vi "checkFinishDeadBallPlayVSS.vi"(8 "error in (no error)":errorcluster, 9 "last command_interpreted":T1, 10 "Game":refnum<class "Game.lvclass">, 11 "DeadBallPlayVSS in":refnum<class "DeadBallPlayVSS.lvclass">) -> (0 "error out":errorcluster, 2 "Boolean":bool, 3 "DeadBallPlayVSS out":refnum<class "DeadBallPlayVSS.lvclass">)   [LabVIEW 2023, in "DeadBallPlayVSS.lvclass"]
uses:
  DeadBallPlayVSS.lvclass
  Game_class/Game.lvclass
  Referee_class/command_interpreted.ctl
  Utilities_class/Utilities.lvclass
  Game_class/Game.lvclass/Game.ctl
  Ball_class/Ball.lvclass/Ball.ctl
  Events_class/Events.lvclass/Events.ctl
  Game_class/Read BallRef.vi
  Game_class/Read EventsRef.vi
  Events_class/Read ball_out.vi
  Events_class/Read ball_out_of_vision.vi
  Ball_class/Read v_x.vi
  Ball_class/Read v_y.vi
  Ball_class/Ball.lvclass
  Events_class/Events.lvclass
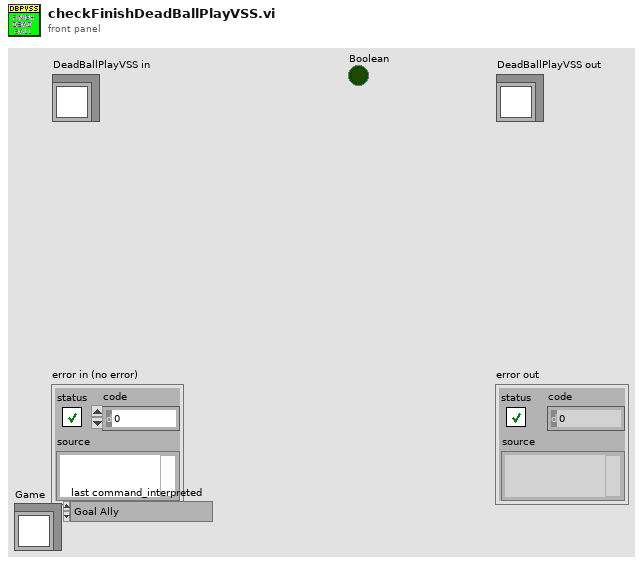
[diagram p1: front panel]
types:
  T1 = typedef "command_interpreted.ctl" = enum16{"Goal Ally", "Goal Enemy", "Ball Placement Enemy", "Ball Placement Ally", "Normal Half Time", "Extra Time  Break", "Extra Half Time", "None", "Post Game", "PKA Normal Start", "Prepare Kickoff Ally", "PKE Normal Start", "Prepare Kickoff Enemy", "Force Start", "Halt", "Timeout", "Prepare Penalty Ally", "Prepare Penalty Enemy", "PPA NormalStart", "PPE Normal Start", "Indirect Free Ally", "Direct Free Enemy", "Direct Free Ally", "Indirect Free Enemy", "Stop"}
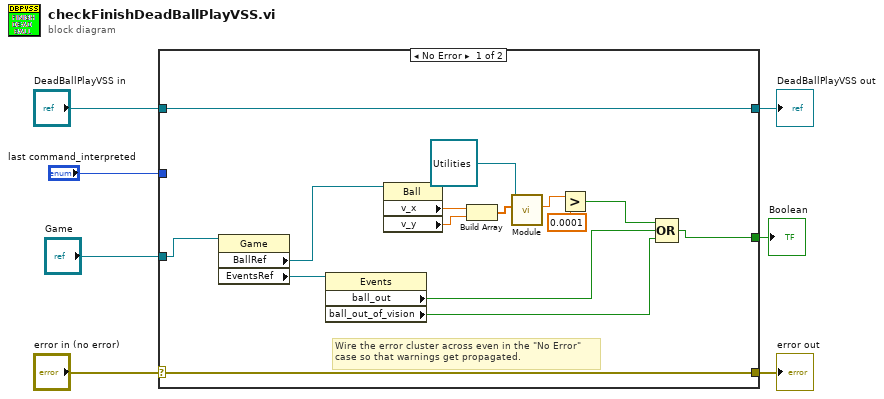
[diagram p0: block diagram]
diagram:
  n1 = case shown="No Error" "error in (no error)" {
    selector: "error in (no error)" -> [w21 w24]
    tunnel: [w21 w24] -> w6
    tunnel: [w22 w23] -> w4
    tunnel: "DeadBallPlayVSS in" -> [w22 w23]
    tunnel: "last command_interpreted" -> [_ _]
    tunnel: "Game" -> [w20 _]
    tunnel: [w8 _] -> w1
    frame No Error {
      # "Wire the error cluster across even in the \"No Error\"\ncase so that warnings get propagated."
      n2 = property class="Game"(reference=w20) -> ("BallRef"=w19:refnum<class "Ball.lvclass">, "EventsRef"=w12:refnum<class "Events.lvclass">)  [unwired: 1 in, 2 out]
      n3 = property class="Events"(reference=w12) -> ("ball_out"=w10:bool, "ball_out_of_vision"=w9:bool)  [unwired: 1 in, 2 out]
      n4 = property class="Ball"(reference=w19) -> ("v_x"=w18:dbl, "v_y"=w17:dbl)  [unwired: 1 in, 2 out]
      n5 = Build Array(w18, w17) -> (w16:dbl[])
      n6 = call-dynamic "Module.vi"("2D vector"=w16, "Utilities in"=refnum<class "Utilities.lvclass"> refnum) -> ("Modulo"=w14:dbl)  [unwired: 7 in, 2 out]
      n7 = Greater?(x=w14, y=0.0001) -> (0:w11:bool)
      n8 = Compound Arithmetic op=OR(w11, w10, w9) -> (w8:bool)
    }
    frame Error {
    }
  }
  "error out" <- w6
  "DeadBallPlayVSS out" <- w4
  "Boolean" <- w1
